vi "Editor Controller.vi"(8 "error in (no error)":errorcluster, 11 "Editor Handler in":refnum<class "Image Editor Handler.lvclass">) -> (0 "error out":errorcluster, 3 "Editor Handler out":refnum<class "Image Editor Handler.lvclass">)   [LabVIEW 2015, in "LV Image Editor Framework.lvlib" / "Image Editor Handler.lvclass"]
uses:
  Image Editor Handler.lvclass
  Image Editor Handler.lvclass/Image Editor Handler.ctl
  Image/Image.lvclass/Image.ctl
  Image/Image.lvclass
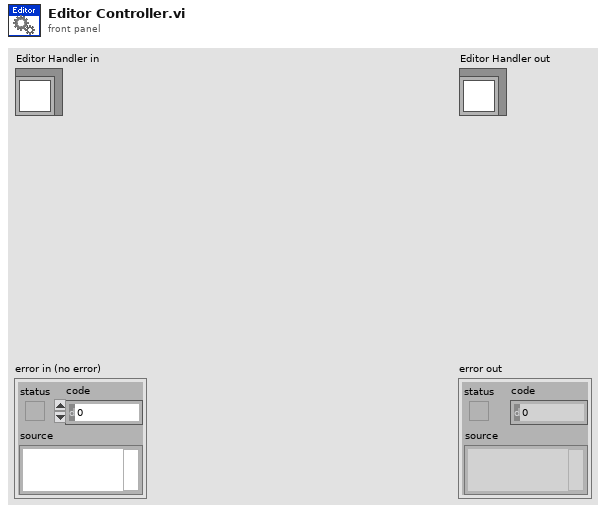
[diagram p1: front panel]
types:
  T1 = typedef "LV Image Editor Framework.lvlib/Image Editor Handler.lvclass/Editor Events.ctl" = cluster{"Stop":refnum<user-event>, "Keyboard Events":cluster{"KeyDown Data":refnum<user-event>, "KeyRepeat Data":refnum<user-event>}, "Mouse Events":cluster{"MouseDown Data":refnum<user-event>, "MouseMove Data":refnum<user-event>, "MouseUp Data":refnum<user-event>}, "Menu Events":cluster{"Shortcut Act Data":refnum<user-event>, "MenuSelection Data":refnum<user-event>}, "Image Events":cluster{"AddShape":refnum<user-event>, "Paint":refnum<user-event>, "RemoveShape":refnum<user-event>, "RefreshShape":refnum<user-event>, "ShapePropertyChange":refnum<user-event>}, "RequestShapes":refnum<user-event>, "Custom":refnum<user-event>}
  T2 = typedef "eventvkey.ctl" = enum16{"ASCII", "Enter", "Return", "Shift", "Ctrl", "Alt", "Cmd", "Opt", "Caps", "NumLock", "Clear", "Break", "Up", "Down", "Left", "Right", "Insert", "Delete", "Home", "End", "PageUp", "PageDown", "Escape", "Help", "Pause", "ScrollLock", "F1", "F2", "F3", "F4", "F5", "F6", "F7", "F8", "F9", "F10", "F11", "F12", "F13", "F14", "F15", "F16", "F17", "F18", "F19", "F20", "F21", "F22", "F23", "F24", "Play", "VolumeUp", "VolumeDown", "Mute", "Two Byte Char"}
  T3 = cluster{"Shift":bool, "Ctrl":bool, "Alt":bool, "Cmd":bool, "Opt":bool}
  T4 = typedef "LVPoint32TypeDef.ctl" = cluster{"Horizontal":i32, "Vertical":i32}
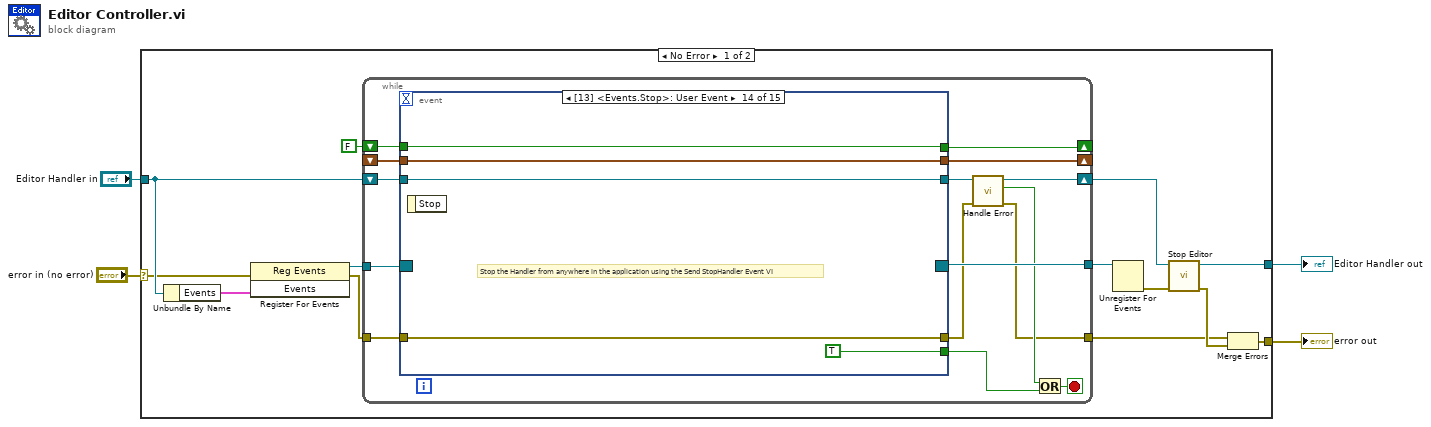
[diagram p0: block diagram]
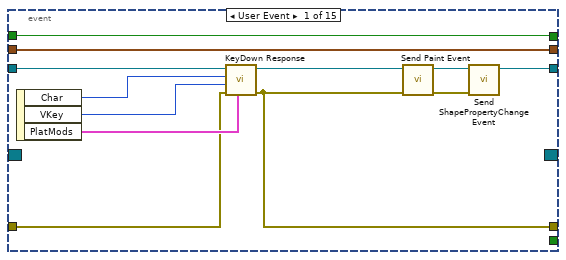
[diagram p2: hidden frame]
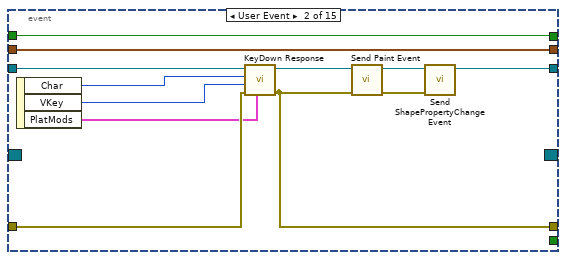
[diagram p3: hidden frame]
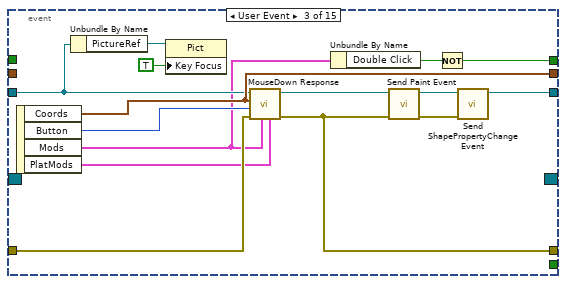
[diagram p4: hidden frame]
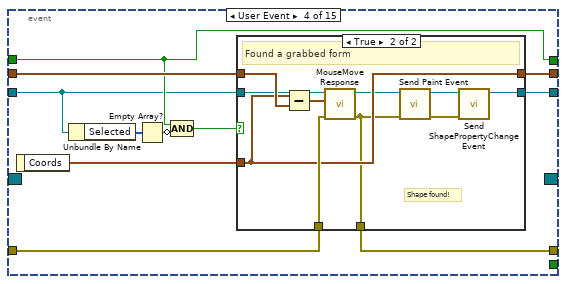
[diagram p5: hidden frame]
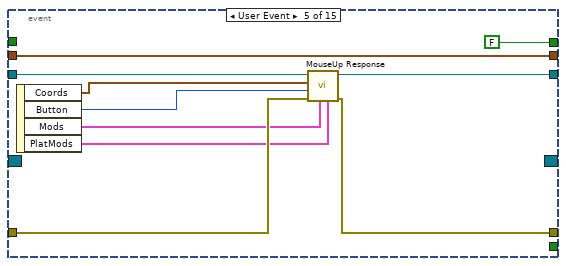
[diagram p7: hidden frame]
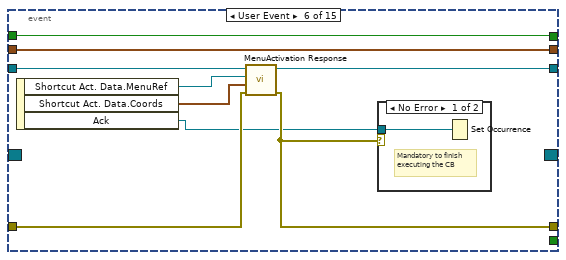
[diagram p8: hidden frame]
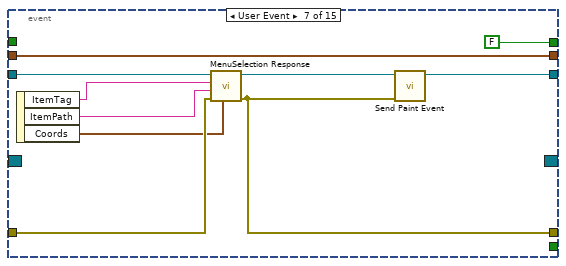
[diagram p10: hidden frame]
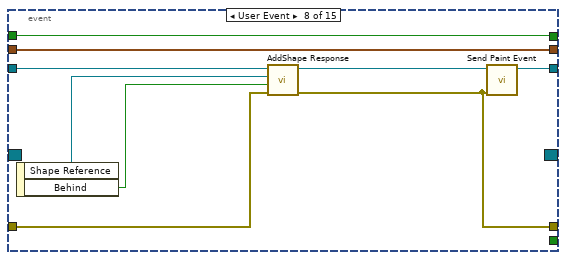
[diagram p11: hidden frame]
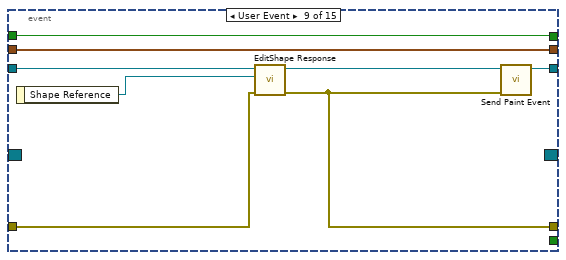
[diagram p12: hidden frame]
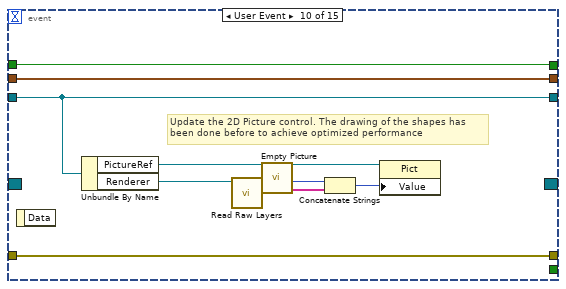
[diagram p13: hidden frame]
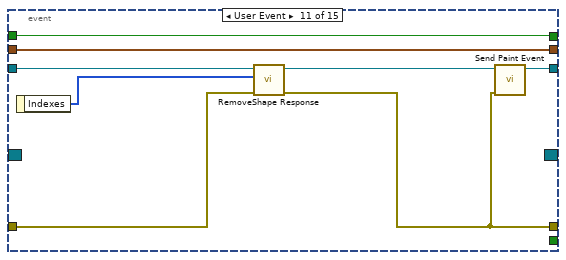
[diagram p14: hidden frame]
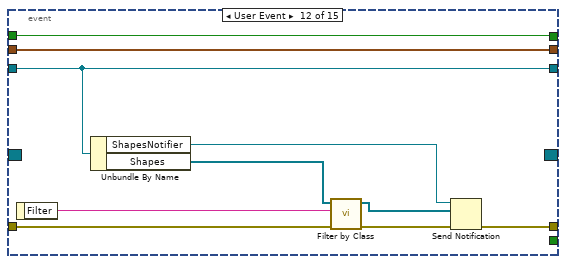
[diagram p15: hidden frame]
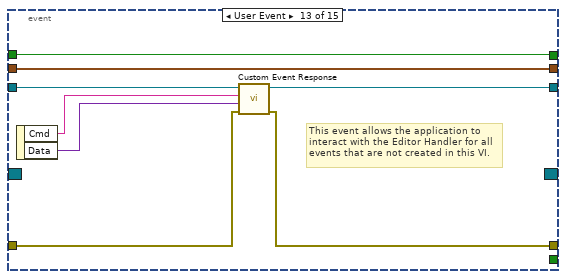
[diagram p16: hidden frame]
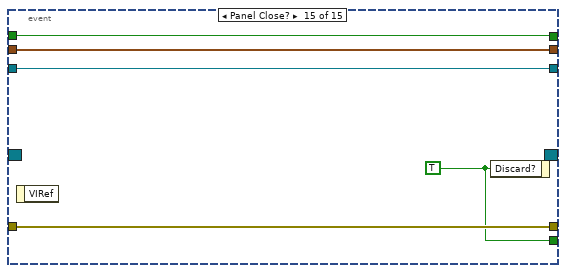
[diagram p17: hidden frame]
diagram:
  n1 = case shown="No Error" "error in (no error)" {
    selector: "error in (no error)" -> [w13 w189]
    tunnel: "Editor Handler in" -> [w17 w188]
    tunnel: [w8 w188] -> w2
    tunnel: [w6 w189] -> w1
    frame No Error {
      n2 = Unbundle By Name(w17) -> ("Events"=w11:T1)
      n3 = register-events(error in=w13, w11) -> (reference out=w16:refnum<event-registration>, error out=w12:errorcluster)  [unwired: 1 in]
      n4 = while {
        tunnel: w16 -> [w24]
        shift-right: [w19] -> w10
        shift-left: w17 -> [w32]
        shift-right: [w29] -> _
        shift-left: _ -> [w28]
        shift-right: [w27] -> _
        shift-left: FALSE -> [w26]
        tunnel: [w25] -> w14
        tunnel: w12 -> [w31]
        tunnel: [w18] -> w5
        stop <- w22 stop-if-true
        n5 = event shown="[13] <Events.Stop>: User Event" {
          selector: w24 -> [_ _ _ _ _ _ _ _ _ _ _ _ _ _ _]
          dyn-events: [_ _ _ _ _ _ _ _ _ _ _ _ _ _ _] -> w25
          timeout: _ -> [_ _ _ _ _ _ _ _ _ _ _ _ _ _ _]
          tunnel: w32 -> [w44 w54 w64 w75 w103 w112 w123 w134 w140 w147 w157 w166 w175 w181 w186]
          tunnel: [w33 w46 w62 w74 w102 w111 w117 w129 w138 w147 w155 w166 w174 w181 w186] -> w20
          tunnel: w31 -> [w40 w53 w70 w72 w100 w110 w124 w127 w136 w143 w154 w163 w171 w182 w187]
          tunnel: [w36 w48 w61 w73 w101 w109 w116 w126 w135 w143 w153 w165 w170 w182 w187] -> w23
          tunnel: [_ _ _ _ _ _ _ _ _ _ _ _ _ TRUE w183] -> w30
          tunnel: [w38 w56 w68 w79 w105 w114 w125 w131 w142 w144 w159 w169 w177 w178 w184] -> w29
          tunnel: w28 -> [w38 w56 _ w81 w105 w114 w125 w131 w142 w144 w159 w169 w177 w178 w184]
          tunnel: [w39 w55 w58 w78 FALSE w113 FALSE w132 w141 w145 w158 w168 w176 w179 w185] -> w27
          tunnel: w26 -> [w39 w55 _ w78 _ w113 _ w132 w141 w145 w158 w168 w176 w179 w185]
          event User Event {
            n6 = event-data() -> ("Char"=w43:i16, "VKey"=w42:T2, "PlatMods"=w41:T3)  [unwired: 1 in]
            n7 = call-dynamic "KeyDown Response.vi"("PlatMods"=w41, "error in (no error)"=w40, "VKey"=w42, "Char"=w43, "Editor Handler in"=w44) -> ("error out"=w36:errorcluster, "Editor Handler out"=w37:refnum<class "Image Editor Handler.lvclass">)  [unwired: 5 in]
            n8 = call "Send Paint Event.vi"("error in (no error)"=w36, "Editor Handler in"=w37) -> ("error out"=w34:errorcluster, "Editor Handler out"=w35:refnum<class "Image Editor Handler.lvclass">)  [unwired: 8 in]
            n9 = call "Send ShapePropertyChange Event.vi"("error in (no error)"=w34, "Editor Handler in"=w35) -> ("Editor Handler out"=w33:refnum<class "Image Editor Handler.lvclass">)  [unwired: 8 in, 1 out]
          }
          event User Event {
            n10 = event-data() -> ("Char"=w51:i16, "VKey"=w50:T2, "PlatMods"=w49:T3)  [unwired: 1 in]
            n11 = call-dynamic "KeyDown Response.vi"("PlatMods"=w49, "error in (no error)"=w53, "VKey"=w50, "Char"=w51, "Editor Handler in"=w54) -> ("error out"=w48:errorcluster, "Editor Handler out"=w52:refnum<class "Image Editor Handler.lvclass">)  [unwired: 5 in]
            n12 = call "Send Paint Event.vi"("error in (no error)"=w48, "Editor Handler in"=w52) -> ("error out"=w45:errorcluster, "Editor Handler out"=w47:refnum<class "Image Editor Handler.lvclass">)  [unwired: 8 in]
            n13 = call "Send ShapePropertyChange Event.vi"("error in (no error)"=w45, "Editor Handler in"=w47) -> ("Editor Handler out"=w46:refnum<class "Image Editor Handler.lvclass">)  [unwired: 8 in, 1 out]
          }
          event User Event {
            n14 = event-data() -> ("Coords"=w68:T4, "Button"=w71:u16, "Mods"=w60:cluster{"Double Click":bool, "Menu Key":bool}, "PlatMods"=w69:T3)  [unwired: 1 in]
            n15 = Unbundle By Name(w64) -> ("PictureRef"=w66:refnum<vi>)
            n16 = property class="Pict"(reference=w66, "Key Focus"=TRUE) -> ()  [unwired: 1 in, 2 out]
            n17 = call-dynamic "MouseDown Response.vi"("PlatMods"=w69, "Mods"=w60, "error in (no error)"=w70, "Button"=w71, "Coords"=w68, "Editor Handler in"=w64) -> ("error out"=w61:errorcluster, "Editor Handler out"=w67:refnum<class "Image Editor Handler.lvclass">)  [unwired: 4 in]
            n18 = Unbundle By Name(w60) -> ("Double Click"=w59:bool)
            n19 = call "Send Paint Event.vi"("error in (no error)"=w61, "Editor Handler in"=w67) -> ("error out"=w57:errorcluster, "Editor Handler out"=w63:refnum<class "Image Editor Handler.lvclass">)  [unwired: 8 in]
            n20 = Not(x=w59) -> (.not. x?=w58:bool)
            n21 = call "Send ShapePropertyChange Event.vi"("error in (no error)"=w57, "Editor Handler in"=w63) -> ("Editor Handler out"=w62:refnum<class "Image Editor Handler.lvclass">)  [unwired: 8 in, 1 out]
          }
          event User Event {
            n22 = event-data() -> ("Coords"=w80:T4)  [unwired: 1 in]
            n23 = Unbundle By Name(w75) -> ("Selected"=w82:i16[])
            n24 = Empty Array?(array=w82) -> (empty?=w77:bool)
            n25 = Compound Arithmetic op=AND(w78, invert w77) -> (w76:bool)
            n26 = case shown="True" w76 {
              tunnel: w81 -> [w85 w95]
              tunnel: w80 -> [_ w91]
              tunnel: [w85 w91] -> w79
              tunnel: w75 -> [w84 w94]
              tunnel: [w84 w87] -> w74
              tunnel: [w83 w90] -> w73
              tunnel: w72 -> [w83 w92]
              frame False {
                # "Note: this event will be triggered very often. Don't add code unless it's crucial"
                # "Do nothing if no shape has been found"
                # "No selected form"
              }
              frame True {
                # "Shape found!"
                # "Found a grabbed form"
                n27 = Subtract(x=w91, y=w95) -> (x-y=w93:T4)
                n28 = call-dynamic "MouseMove Response.vi"("error in (no error)"=w92, "Delta"=w93, "Editor Handler in"=w94) -> ("error out"=w90:errorcluster, "Editor Handler out"=w89:refnum<class "Image Editor Handler.lvclass">)  [unwired: 7 in]
                n29 = call "Send Paint Event.vi"("error in (no error)"=w90, "Editor Handler in"=w89) -> ("error out"=w86:errorcluster, "Editor Handler out"=w88:refnum<class "Image Editor Handler.lvclass">)  [unwired: 8 in]
                n30 = call "Send ShapePropertyChange Event.vi"("error in (no error)"=w86, "Editor Handler in"=w88) -> ("Editor Handler out"=w87:refnum<class "Image Editor Handler.lvclass">)  [unwired: 8 in, 1 out]
              }
            }
          }
          event User Event {
            n31 = event-data() -> ("Coords"=w99:T4, "Button"=w98:u16, "Mods"=w97:cluster{"Double Click":bool, "Menu Key":bool}, "PlatMods"=w96:T3)  [unwired: 1 in]
            n32 = call-dynamic "MouseUp Response.vi"("PlatMods"=w96, "Mods"=w97, "error in (no error)"=w100, "Button"=w98, "Coords"=w99, "Editor Handler in"=w103) -> ("error out"=w101:errorcluster, "Editor Handler out"=w102:refnum<class "Image Editor Handler.lvclass">)  [unwired: 4 in]
          }
          event User Event {
            n33 = event-data() -> ("Shortcut Act. Data.MenuRef"=w108:refnum<k9>, "Shortcut Act. Data.Coords"=w107:T4, "Ack"=w106:refnum<k4>)  [unwired: 1 in]
            n34 = call-dynamic "MenuActivation Response.vi"("error in (no error)"=w110, "Coords"=w107, "Menu Refnum"=w108, "Editor Handler in"=w112) -> ("error out"=w109:errorcluster, "Editor Handler out"=w111:refnum<class "Image Editor Handler.lvclass">)  [unwired: 6 in]
            n35 = case shown="No Error" w109 {
              tunnel: w106 -> [w115 _]
              frame No Error {
                # "Mandatory to finish executing the CB"
                n36 = Set Occurrence(w115) -> ()
              }
              frame Error {
              }
            }
          }
          event User Event {
            n37 = event-data() -> ("ItemTag"=w121:string, "ItemPath"=w120:string, "Coords"=w119:T4)  [unwired: 1 in]
            n38 = call-dynamic "MenuSelection Response.vi"("Coords"=w119, "error in (no error)"=w124, "Menu Name"=w120, "Menu Tag"=w121, "Editor Handler in"=w123) -> ("error out"=w116:errorcluster, "Editor Handler out"=w118:refnum<class "Image Editor Handler.lvclass">)  [unwired: 5 in]
            n39 = call "Send Paint Event.vi"("error in (no error)"=w116, "Editor Handler in"=w118) -> ("Editor Handler out"=w117:refnum<class "Image Editor Handler.lvclass">)  [unwired: 8 in, 1 out]
          }
          event User Event {
            n40 = event-data() -> ("Shape Reference"=w133:refnum<data-value>, "Behind"=w128:bool)  [unwired: 1 in]
            n41 = call-dynamic "AddShape Response.vi"("error in (no error)"=w127, "Behind"=w128, "Shape Reference"=w133, "Image Editor Handler in"=w134) -> ("error out"=w126:errorcluster, "Image Editor Handler out"=w130:refnum<class "Image Editor Handler.lvclass">)  [unwired: 6 in]
            n42 = call "Send Paint Event.vi"("error in (no error)"=w126, "Editor Handler in"=w130) -> ("Editor Handler out"=w129:refnum<class "Image Editor Handler.lvclass">)  [unwired: 8 in, 1 out]
          }
          event User Event {
            n43 = event-data() -> ("Shape Reference"=w137:refnum<data-value>)  [unwired: 1 in]
            n44 = call "EditShape Response.vi"("error in (no error)"=w136, "Shape Reference"=w137, "Editor Handler in"=w140) -> ("error out"=w135:errorcluster, "Editor Handler out"=w139:refnum<class "Image Editor Handler.lvclass">)  [unwired: 7 in]
            n45 = call "Send Paint Event.vi"("error in (no error)"=w135, "Editor Handler in"=w139) -> ("Editor Handler out"=w138:refnum<class "Image Editor Handler.lvclass">)  [unwired: 8 in, 1 out]
          }
          event User Event {
            # "Update the 2D Picture control. The drawing of the shapes has been done before to achieve optimized performance"
            n46 = event-data() -> ()  [unwired: 1 in, 1 out]
            n47 = Unbundle By Name(w147) -> ("PictureRef"=w146:refnum<vi>, "Renderer"=w151:refnum<class "Image.lvclass">)
            n48 = call "Read Raw Layers.vi"("Image in"=w151) -> ("Raw Layers"=w150:string[])  [unwired: 9 in, 1 out]
            n49 = call "Empty Picture"() -> ("empty picture"=w149:picture)
            n50 = Concatenate Strings(w149, w150) -> (w148:picture)
            n51 = property class="Pict"(reference=w146, "Value"=w148) -> ()  [unwired: 1 in, 2 out]
          }
          event User Event {
            n52 = event-data() -> ("Indexes"=w152:i32[])  [unwired: 1 in]
            n53 = call-dynamic "RemoveShape Response.vi"("error in (no error)"=w154, "Indexes"=w152, "Image Editor Handler in"=w157) -> ("error out"=w153:errorcluster, "Image Editor Handler out"=w156:refnum<class "Image Editor Handler.lvclass">)  [unwired: 7 in]
            n54 = call "Send Paint Event.vi"("error in (no error)"=w153, "Editor Handler in"=w156) -> ("Editor Handler out"=w155:refnum<class "Image Editor Handler.lvclass">)  [unwired: 8 in, 1 out]
          }
          event User Event {
            n55 = event-data() -> ("Filter"=w160:string)  [unwired: 1 in]
            n56 = Unbundle By Name(w166) -> ("ShapesNotifier"=w167:refnum<notifier>, "Shapes"=w161:refnum<data-value>[])
            n57 = call "Filter by Class.vi"("error in (no error)"=w163, "Filter"=w160, "Shapes in"=w161) -> ("error out"=w162:errorcluster, "Shapes out"=w164:refnum<data-value>[])  [unwired: 7 in]
            n58 = Send Notification(notification=w164, notifier=w167, error in (no error)=w162) -> (error out=w165:errorcluster)  [unwired: 1 out]
          }
          event User Event {
            # "This event allows the application to interact with the Editor Handler for all events that are not created in this VI."
            n59 = event-data() -> ("Cmd"=w173:string, "Data"=w172:variant)  [unwired: 1 in]
            n60 = call-dynamic "Custom Event Response.vi"("error in (no error)"=w171, "Data"=w172, "Cmd"=w173, "Image Editor Handler in"=w175) -> ("error out"=w170:errorcluster, "Image Editor Handler out"=w174:refnum<class "Image Editor Handler.lvclass">)  [unwired: 6 in]
          }
          event User Event {
            # "Stop the Handler from anywhere in the application using the Send StopHandler Event VI"
            n61 = event-data() -> ()  [unwired: 1 in, 1 out]
          }
          event Panel Close? {
            w183 = TRUE ("Discard?")
            n62 = event-data() -> ()  [unwired: 1 in, 1 out]
            n63 = event-data("Discard?"=w183) -> ()  [unwired: 1 in, 1 out]
          }
        }
        n64 = call-dynamic "Handle Error.vi"("error in (no error)"=w23, "Image Editor Handler in"=w20) -> ("error out"=w18:errorcluster, "Stop Controller"=w21:bool, "Image Editor Handler out"=w19:refnum<class "Image Editor Handler.lvclass">)  [unwired: 7 in]
        n65 = Or(x=w21, y=w30) -> (x .or. y?=w22:bool)
      }
      n66 = Unregister For Events(event registration refnum=w14) -> (error out=w9:errorcluster)  [unwired: 1 in]
      n67 = call-dynamic "Stop Editor.vi"("error in (no error)"=w9, "Editor Handler in"=w10) -> ("error out"=w7:errorcluster, "Editor Handler out"=w8:refnum<class "Image Editor Handler.lvclass">)  [unwired: 8 in]
      n68 = Merge Errors(w5, w7) -> (w6:errorcluster)
    }
    frame Error {
    }
  }
  "error out" <- w1
  "Editor Handler out" <- w2
